vi "Abort Read.vi"() -> ()   [LabVIEW 2020]
panel:
  in  "Abort Read":bool
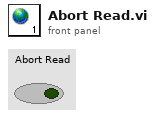
[diagram p1: front panel]
diagram:
